vi "Get Last Err wrapper.vi"(8 "error in (no error)":errorcluster caption="错误输入（无错误）", 10 "dwLen":u32, 11 "ErrMsg":string) -> (0 "error out":errorcluster caption="错误输出", 2 "function return":u32, 3 "ErrMsg out":string)   [LabVIEW 2016, in "UISimCanFunc_wrapper.lvlib"]
doc: "_declspec (dllexport) DWORD GetLastErr_wrapper(char *ErrMsg, DWORD dwLen);"
uses:
  <userlib>/UISimCanFunc_wrapper/UISimCanFunc_wrapper.lvlib
  <userlib>/UISimCanFunc_wrapper/UISimCanFunc_wrapper.dll
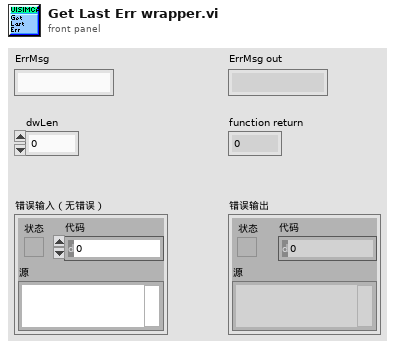
[diagram p1: front panel]
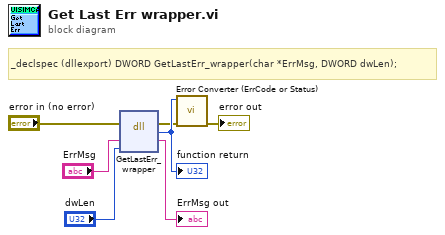
[diagram p0: block diagram]
diagram:
  # "_declspec (dllexport) DWORD GetLastErr_wrapper(char *ErrMsg, DWORD dwLen);"
  n1 = dll-call lib="C:/Program Files (x86)/National Instruments/LabVIEW 2016/user.lib/UISimCanFunc_wrapper/UISimCanFunc_wrapper.*" fn="GetLastErr_wrapper"(error in="error in (no error)", "ErrMsg"="ErrMsg", "dwLen"="dwLen") -> (error out=w2:errorcluster, w7:u32, "ErrMsg"=→"ErrMsg out":string)  [unwired: 3 in, 1 out]
  "function return" <- w7
  n2 = call <userlib>:"Error Converter (ErrCode or Status).vi"("error in (no error)"=w2, "error code"=w7) -> ("error out"=→"error out":errorcluster)  [unwired: 9 in]
